vi "Configure Module.vi"(8 "error in":errorcluster, 10 "IOV ref in":variant, 11 "9216 in":refnum<class "9216.lvclass">) -> (0 "error out":errorcluster, 2 "IOV ref out":variant, 3 "9216 out":refnum<class "9216.lvclass">)   [LabVIEW 2019, in "Modules.lvlib" / "9216.lvclass"]
uses:
  9216.lvclass
  <resource>/objmgr/cRIO.rc
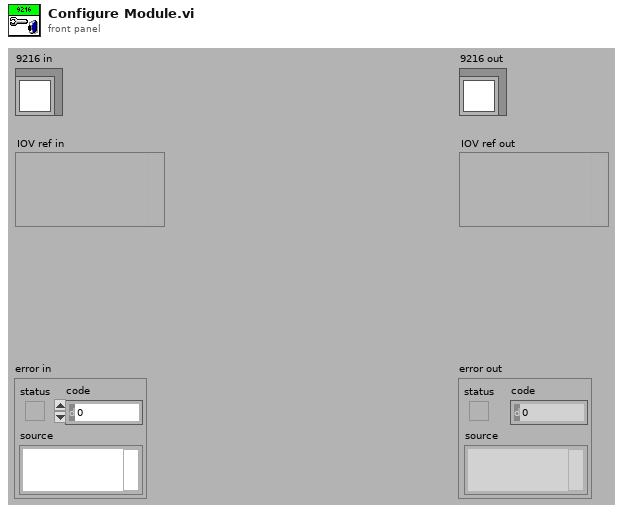
[diagram p1: front panel]
types:
  T1 = cluster{"Ohm degree range":u32, "RTD type":u32, "RTD user-defined A constant":dbl, "RTD user-defined B constant":dbl, "RTD user-defined C constant":dbl, "RTD user-defined Ro constant":dbl}[]
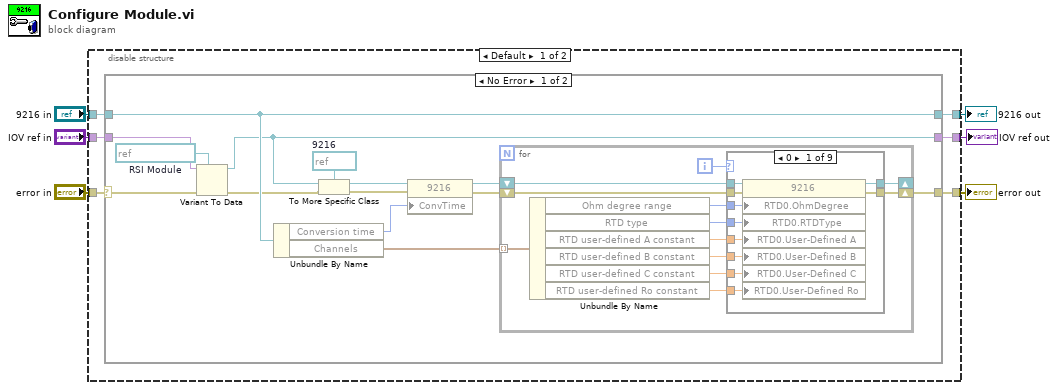
[diagram p0: block diagram]
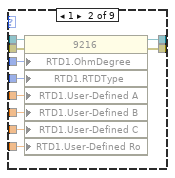
[diagram p2: hidden frame]
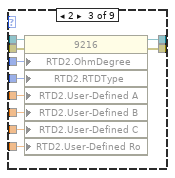
[diagram p3: hidden frame]
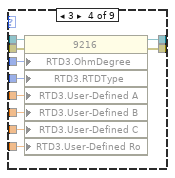
[diagram p4: hidden frame]
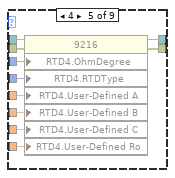
[diagram p5: hidden frame]
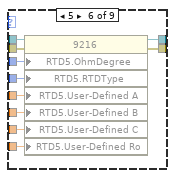
[diagram p6: hidden frame]
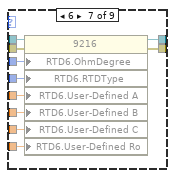
[diagram p7: hidden frame]
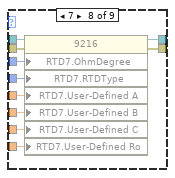
[diagram p8: hidden frame]
diagram:
  n1 = disable-structure shown="Default" {
    disable-tunnel: "error in" -> [w12 w126]
    disable-tunnel: [w11 w126] -> w5
    disable-tunnel: "9216 in" -> [w10 w124]
    disable-tunnel: [w9 w124] -> w3
    disable-tunnel: "IOV ref in" -> [w8 w125]
    disable-tunnel: [w7 w125] -> w1
    frame condition #0 {
      n2 = case shown="No Error" w12 {
        selector: w12 -> [w17 w123]
        tunnel: [w24 w123] -> w11
        tunnel: [w26 w122] -> w9
        tunnel: w10 -> [w26 w122]
        tunnel: w8 -> [w15 w121]
        tunnel: [w14 w121] -> w7
        frame No Error {
          w13 = refnum<k21> refnum  # RSI Module
          w25 = refnum<k21> refnum  # 9216
          n3 = Variant To Data(error in=w17, type=w13, Variant=w15) -> (data=w14:refnum<k21>, error out=w16:errorcluster)
          n4 = Unbundle By Name(w26) -> ("Conversion time"=w23:u16, "Channels"=w18:T1)
          n5 = To More Specific Class(target class=w25, reference=w14, error in=w16) -> (specific class reference=w22:refnum<k21>, error out=w21:errorcluster)
          n6 = property class="9216"(reference=w22, error in=w21, "ConvTime"=w23) -> (reference out=w19:refnum<k21>, error out=w20:errorcluster)
          n7 = for {
            shift-right: [w38] -> w24
            shift-left: w20 -> [w31]
            shift-right: [w29] -> _
            shift-left: w19 -> [w30]
            tunnel: w18 -> [w28] mode=indexing
            i -> [w27]
            n8 = Unbundle By Name(w28) -> ("Ohm degree range"=w37:u32, "RTD type"=w36:u32, "RTD user-defined A constant"=w35:dbl, "RTD user-defined B constant"=w34:dbl, "RTD user-defined C constant"=w33:dbl, "RTD user-defined Ro constant"=w32:dbl)
            n9 = case shown="0" w27 {
              tunnel: [w48 w58 w68 w78 w88 w98 w108 w118 w119] -> w38
              tunnel: w37 -> [w47 w57 w67 w77 w87 w97 w107 w117 _]
              tunnel: w36 -> [w46 w49 w59 w69 w83 w89 w99 w109 _]
              tunnel: w35 -> [w45 w50 w60 w70 w82 w90 w100 w110 _]
              tunnel: w34 -> [w44 w51 w61 w71 w81 w91 w101 w111 _]
              tunnel: w33 -> [w43 w52 w62 w72 w80 w92 w102 w112 _]
              tunnel: w32 -> [w42 w53 w63 w73 w79 w93 w103 w113 _]
              tunnel: w31 -> [w41 w56 w66 w76 w86 w96 w106 w116 w119]
              tunnel: w30 -> [w40 w55 w65 w75 w85 w95 w105 w115 w120]
              tunnel: [w39 w54 w64 w74 w84 w94 w104 w114 w120] -> w29
              frame 0 {
                n10 = property class="9216"(reference=w40, error in=w41, "RTD0.OhmDegree"=w47, "RTD0.RTDType"=w46, "RTD0.User-Defined A"=w45, "RTD0.User-Defined B"=w44, "RTD0.User-Defined C"=w43, "RTD0.User-Defined Ro"=w42) -> (reference out=w39:refnum<k21>, error out=w48:errorcluster)
              }
              frame 1 {
                n11 = property class="9216"(reference=w55, error in=w56, "RTD1.OhmDegree"=w57, "RTD1.RTDType"=w49, "RTD1.User-Defined A"=w50, "RTD1.User-Defined B"=w51, "RTD1.User-Defined C"=w52, "RTD1.User-Defined Ro"=w53) -> (reference out=w54:refnum<k21>, error out=w58:errorcluster)
              }
              frame 2 {
                n12 = property class="9216"(reference=w65, error in=w66, "RTD2.OhmDegree"=w67, "RTD2.RTDType"=w59, "RTD2.User-Defined A"=w60, "RTD2.User-Defined B"=w61, "RTD2.User-Defined C"=w62, "RTD2.User-Defined Ro"=w63) -> (reference out=w64:refnum<k21>, error out=w68:errorcluster)
              }
              frame 3 {
                n13 = property class="9216"(reference=w75, error in=w76, "RTD3.OhmDegree"=w77, "RTD3.RTDType"=w69, "RTD3.User-Defined A"=w70, "RTD3.User-Defined B"=w71, "RTD3.User-Defined C"=w72, "RTD3.User-Defined Ro"=w73) -> (reference out=w74:refnum<k21>, error out=w78:errorcluster)
              }
              frame 4 {
                n14 = property class="9216"(reference=w85, error in=w86, "RTD4.OhmDegree"=w87, "RTD4.RTDType"=w83, "RTD4.User-Defined A"=w82, "RTD4.User-Defined B"=w81, "RTD4.User-Defined C"=w80, "RTD4.User-Defined Ro"=w79) -> (reference out=w84:refnum<k21>, error out=w88:errorcluster)
              }
              frame 5 {
                n15 = property class="9216"(reference=w95, error in=w96, "RTD5.OhmDegree"=w97, "RTD5.RTDType"=w89, "RTD5.User-Defined A"=w90, "RTD5.User-Defined B"=w91, "RTD5.User-Defined C"=w92, "RTD5.User-Defined Ro"=w93) -> (reference out=w94:refnum<k21>, error out=w98:errorcluster)
              }
              frame 6 {
                n16 = property class="9216"(reference=w105, error in=w106, "RTD6.OhmDegree"=w107, "RTD6.RTDType"=w99, "RTD6.User-Defined A"=w100, "RTD6.User-Defined B"=w101, "RTD6.User-Defined C"=w102, "RTD6.User-Defined Ro"=w103) -> (reference out=w104:refnum<k21>, error out=w108:errorcluster)
              }
              frame 7 {
                n17 = property class="9216"(reference=w115, error in=w116, "RTD7.OhmDegree"=w117, "RTD7.RTDType"=w109, "RTD7.User-Defined A"=w110, "RTD7.User-Defined B"=w111, "RTD7.User-Defined C"=w112, "RTD7.User-Defined Ro"=w113) -> (reference out=w114:refnum<k21>, error out=w118:errorcluster)
              }
              frame Default {
              }
            }
          }
        }
        frame Error {
        }
      }
    }
    frame condition #1 (active) {
    }
  }
  "error out" <- w5
  "9216 out" <- w3
  "IOV ref out" <- w1
